vi "Actor Core.vi"(8 "error in":errorcluster, 11 "Stage in":refnum<class "Stage_panel.lvclass">) -> (0 "error out":errorcluster, 3 "Actor out":refnum<class "Actor.lvclass">)   [LabVIEW 2015, in "Stage_panel.lvclass"]
doc: "(<B>Filename</B>: Actor Framework.lvlib:Actor.lvclass:Actor Core.vi)\n\nReceives messages to the actor, reacts to them, and initiates any error handling that may shut the actor down.\n\nDescendant classes may override this VI to append parallel tasks for the actor to complete while it handles messages. Overrides use the Call Parent Method node."
uses:
  Stage_panel.lvclass
  <vilib>/ActorFramework/Actor/Actor.lvclass
  UI/panel_class/panel.lvclass/panel.ctl
  UI/panel_class/panel.lvclass
panel:
  # "Default Stage"
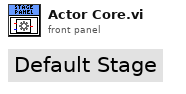
[diagram p1: front panel]
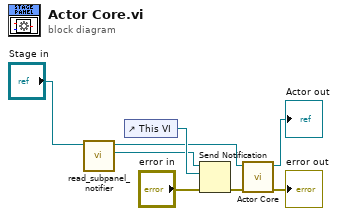
[diagram p0: block diagram]
diagram:
  n1 = call "read_subpanel_notifier.vi"("panel in"="Stage in") -> ("subpanel_notifier"=w1:refnum<notifier>, "panel out"=w2:refnum<class "Stage_panel.lvclass">)  [unwired: 8 in, 1 out]
  n2 = control-ref of="This VI"() -> (w8:refnum<vi>)
  n3 = Send Notification(notification=w8, notifier=w1, error in (no error)="error in") -> (error out=w6:errorcluster)  [unwired: 1 out]
  n4 = call-parent "Actor Core.vi"("error in"=w6, "Actor in"=w2) -> ("error out"=→"error out":errorcluster, "Actor out"=→"Actor out":refnum<class "Actor.lvclass">)  [unwired: 8 in]
